vi "WaveIO-Device Name to ID.vi"(0 "Direction (Input)":u16(ring)=1 items=["Input", "Output", "Loopback", "ASIO input", "ASIO output"], 7 "Device Name":string, 11 "error in (no error)":errorcluster) -> (8 "Device ID":i32=-1, 15 "error out":errorcluster)   [LabVIEW 2020]
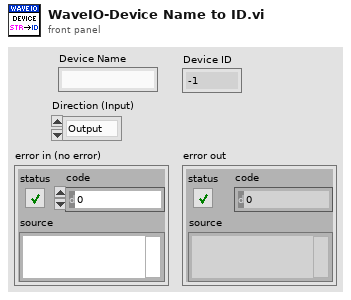
[diagram p1: front panel]
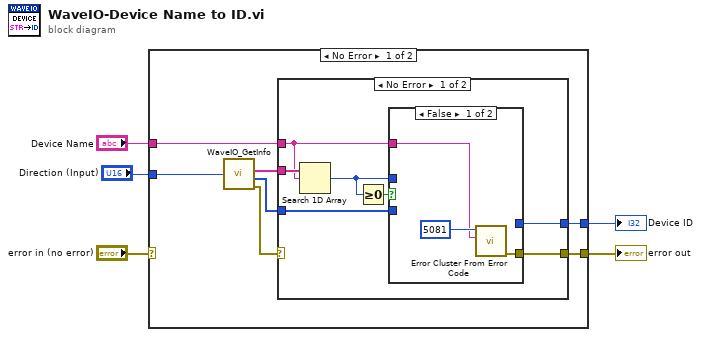
[diagram p0: block diagram]
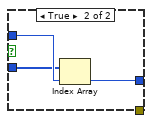
[diagram p2: hidden frame]
diagram:
  n1 = case shown="No Error" "error in (no error)" {
    selector: "error in (no error)" -> [_ w27]
    tunnel: [w12 _] -> w5
    tunnel: "Device Name" -> [w10 _]
    tunnel: [w7 w27] -> w2
    tunnel: "Direction (Input)" -> [w6 _]
    frame No Error {
      n2 = call <userlib>:"WaveIO_GetInfo.vi"("Direction (Input)"=w6) -> ("Dev Names"=w9:string[], "IDDev"=w11:i32[], "error out"=w8:errorcluster)  [unwired: 1 out]
      n3 = case shown="No Error" w8 {
        selector: w8 -> [_ w26]
        tunnel: [w19 _] -> w12
        tunnel: w11 -> [w18 _]
        tunnel: w10 -> [w13 _]
        tunnel: w9 -> [w17 _]
        tunnel: [w14 w26] -> w7
        frame No Error {
          n4 = Search 1D Array(1D array=w17, element=w13) -> (index of element=w15:i32)  [unwired: 1 in]
          n5 = Greater Or Equal To 0?(x=w15) -> (x >= 0?=w16:bool)
          n6 = case shown="False" w16 {
            tunnel: [_ w25] -> w19
            tunnel: w15 -> [_ w24]
            tunnel: w18 -> [_ w23]
            tunnel: [w22 _] -> w14
            tunnel: w13 -> [w20 _]
            frame False {
              n7 = call <vilib>:"Error Cluster From Error Code.vi"("error message (\"\")"=w20, "error code (0)"=5081) -> ("error out"=w22:errorcluster)  [unwired: 7 in]
            }
            frame True {
              n8 = Index Array(array=w23, index=w24) -> (element=w25:i32)
            }
          }
        }
        frame Error {
        }
      }
    }
    frame Error {
    }
  }
  "Device ID" <- w5
  "error out" <- w2
